vi "TCP Factory Wrapper.vi"(8 "error in (no error)":errorcluster, 10 "TCP settings":T1) -> (0 "error out":errorcluster, 3 "TCP out":refnum<class "TCP.lvclass">)   [LabVIEW 2018, in "Instrument Addon Scripting API.lvlib"]
uses:
  Instrument Addon Scripting API.lvlib
  Addon/Support Libraries/Protocols.lvlibp/TCP/TCP Settings.ctl
  Addon/Support Libraries/Protocols.lvlibp/TCP/TCP.lvclass
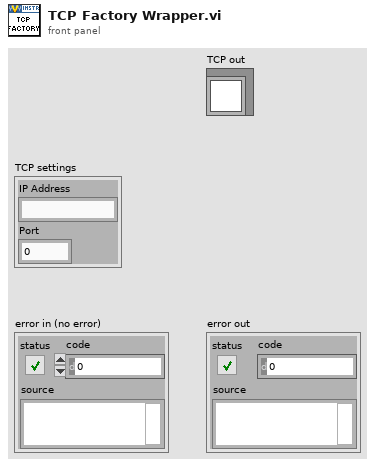
[diagram p1: front panel]
types:
  T1 = typedef "Protocols.lvlibp/TCP.lvclass/TCP Settings.ctl" = cluster{"IP Address":string, "Port":u16}
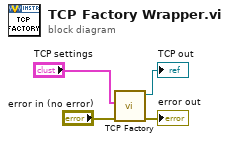
[diagram p0: block diagram]
diagram:
  n1 = call "TCP Factory.vi"("Error In"="error in (no error)", "TCP Settings"="TCP settings") -> ("Error Out"=→"error out":errorcluster, "TCP Out"=→"TCP out":refnum<class "TCP.lvclass">)  [unwired: 8 in]
